vi "Create Generic Queues.vi"(8 "error in (no error)":errorcluster, 11 "name":string="selectspectrum") -> (0 "error out":errorcluster, 3 "Message Queues":T1)   [LabVIEW 2023, in "Front Panel Message Queue.lvlib"]
doc: "This VI creates and initializes all the message queues for your application. If your application requires more than one message queue, right-click the \"Message Queues\" constant above and select Open Type Def. Add the new Message Queue(s) to the type definition, then initialize them in this VI."
uses:
  Front Panel Message Queue.lvlib
  load Message Queues.ctl
  Message Cluster.ctl
  selspectrum Message Queues.ctl
  Enqueue Message (Single).vi
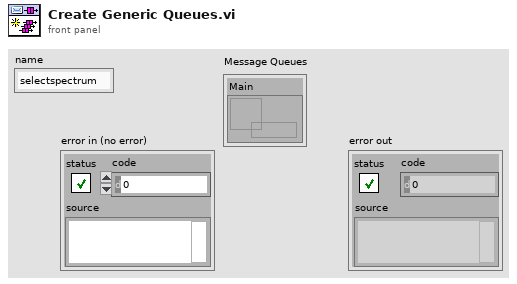
[diagram p1: front panel]
types:
  T1 = typedef "Front Panel Message Queue.lvlib/load Message Queues.ctl" = cluster{"Main":refnum<queue>}
  T2 = typedef "Front Panel Message Queue.lvlib/selspectrum Message Queues.ctl" = cluster{"Main":refnum<queue>}
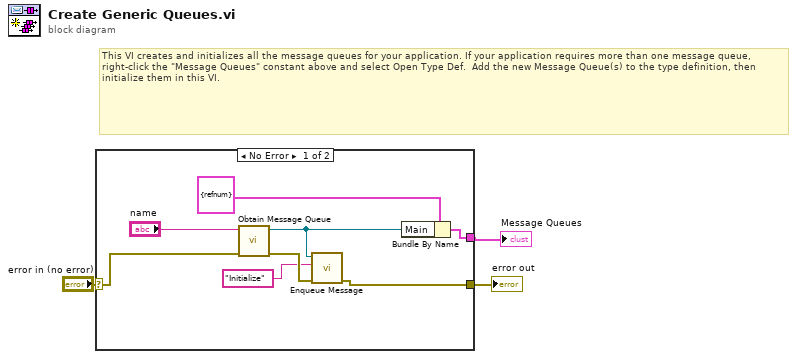
[diagram p0: block diagram]
diagram:
  # "This VI creates and initializes all the message queues for your application. If your application requires more than one message queue, right-click the \"Message Queues\" constant above and select Open Type Def.  Add the new Message Queue(s) to the type definition, then initialize them in this VI."
  n1 = case shown="No Error" "error in (no error)" {
    selector: "error in (no error)" -> [w7 w12]
    tunnel: [w8 w12] -> w3
    tunnel: [w11 _] -> w1
    frame No Error {
      n2 = call "Obtain Message Queue.vi"("error in (no error)"=w7, "name"="name") -> ("error out"=w10:errorcluster, "Message Queue"=w9:refnum<queue>)  [unwired: 8 in]
      n3 = call-poly "Enqueue Message.vi"("error in (no error)"=w10, "Message"="Initialize", "Message Queue"=w9) -> ("error out"=w8:errorcluster)  [unwired: 7 in, 1 out]
      n4 = Bundle By Name(cluster=T2 {"Main"=refnum} ("Message Queues"), "Main"=w9) -> (w11:T2)
    }
    frame Error {
    }
  }
  "error out" <- w3
  "Message Queues" <- w1
